vi "XML ( Prefix_Handler ).vi"(11 "input string":string) -> (3 "result string":string)   [LabVIEW 2018, in "XML.lvlib" / "XML.lvclass"]
uses:
  XML.lvclass
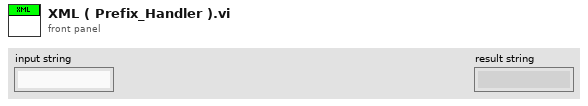
[diagram p1: front panel]
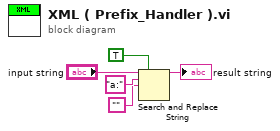
[diagram p0: block diagram]
diagram:
  n1 = Search and Replace String(replace all?=TRUE ("replace all? (F)"), input string="input string", search string="a:", replace string="" ("Namespace Prefix")) -> (result string=→"result string":string)  [unwired: 4 in, 3 out]
